vi "Utility_X-Y Graphs for ROI.vi"(7 "Graphing Action":enum16{"Clear", "Append", "Get"}(ring), 8 "error in (no error)":errorcluster, 9 "Data":dbl[](array[numeric]), 10 "LIMLOCALMETADATA":T1 {"dTimeMSec" format="%.2f"}) -> (0 "error out":errorcluster, 2 "Graph Out":cluster{"X":dbl[], "Y":dbl[]}[](array[cluster]))   [LabVIEW 2014]
uses:
  ND2_Reader_32bit/controls/cluster_LIMLOCALMETADATA.ctl
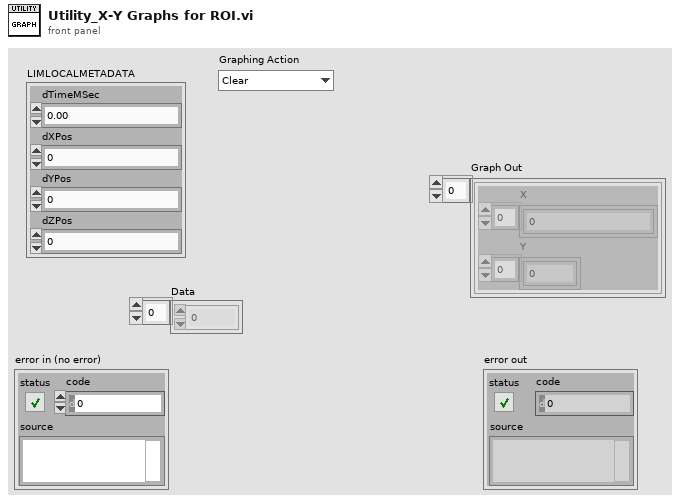
[diagram p1: front panel]
types:
  T1 = typedef "cluster_LIMLOCALMETADATA.ctl" = cluster{"dTimeMSec":dbl, "dXPos":dbl, "dYPos":dbl, "dZPos":dbl}
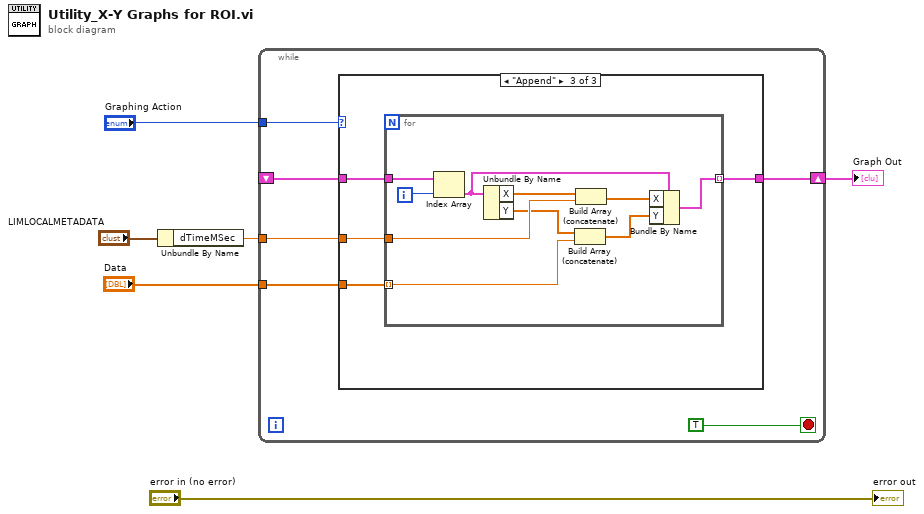
[diagram p0: block diagram]
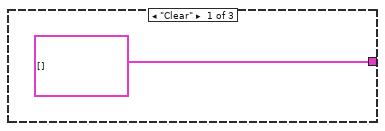
[diagram p2: hidden frame]
diagram:
  n1 = Unbundle By Name("LIMLOCALMETADATA") -> ("dTimeMSec"=w1:dbl)
  n2 = while {
    shift-right: [w10] -> w4
    shift-left: _ -> [w9]
    tunnel: "Graphing Action" -> [w11]
    tunnel: "Data" -> [w8]
    tunnel: w1 -> [w7]
    stop <- TRUE stop-if-true
    n3 = case shown="\"Append\"" w11 {
      tunnel: [cluster{"X":dbl[], "Y":dbl[]}[] [] ("Graph Out") w14 w15] -> w10
      tunnel: w9 -> [_ w14 w18]
      tunnel: w8 -> [_ _ w17]
      tunnel: w7 -> [_ _ w16]
      frame "Clear" {
      }
      frame "Get" {
      }
      frame "Append" {
        n4 = for {
          tunnel: w18 -> [w28]
          tunnel: w17 -> [w22] mode=indexing
          tunnel: w16 -> [w24]
          tunnel: [w19] -> w15 mode=indexing
          i -> [w27]
          n5 = Index Array(array=w28, index=w27) -> (element=w25:cluster{"X":dbl[], "Y":dbl[]})
          n6 = Unbundle By Name(w25) -> ("X"=w26:dbl[], "Y"=w23:dbl[])
          n7 = Build Array (concatenate)(w23, w22) -> (w20:dbl[])
          n8 = Build Array (concatenate)(w26, w24) -> (w21:dbl[])
          n9 = Bundle By Name(cluster=w25, "X"=w21, "Y"=w20) -> (w19:cluster{"X":dbl[], "Y":dbl[]})
        }
      }
    }
  }
  "Graph Out" <- w4
  "error out" <- "error in (no error)"
